vi "capture.vi"() -> ()   [LabVIEW 2014]
uses:
  <vilib>/Instr/_visa.llb/VISA Configure Serial Port (Instr).vi
panel:
  in  "stop":bool
  in  "Home":bool
  in  "error in (no error)":errorcluster
  in  "stop 2":bool
  out "x-position":dbl
  out "y-position":dbl
  out "z-position":dbl
  in  "X um":dbl
  in  "Y um":dbl
  out "error out":errorcluster
  in  "VISA resource name":refnum<visa-resource-name>
  out "y":sgl
  out "x":sgl
  out "Coordinate System Out (Set Coordinate System 1)":T1 {"Measurement System"."Axis Reference" items=["Direct", "Indirect"]; "Measurement System"."Angle (deg)" format="%.2f"; "Measurement System"."Origin"."Y" format="%.2f"; "Measurement System"."Origin"."X" format="%.2f"; "Reference System"."Axis Reference" items=["Direct", "Indirect"]; "Reference System"."Angle (deg)" format="%.2f"; "Reference System"."Origin"."Y" format="%.2f"; "Reference System"."Origin"."X" format="%.2f"}
  out "Objects (pixel) (Object Tracking 1)":T2(array[cluster])
  out "Image":T3(plugin-control)
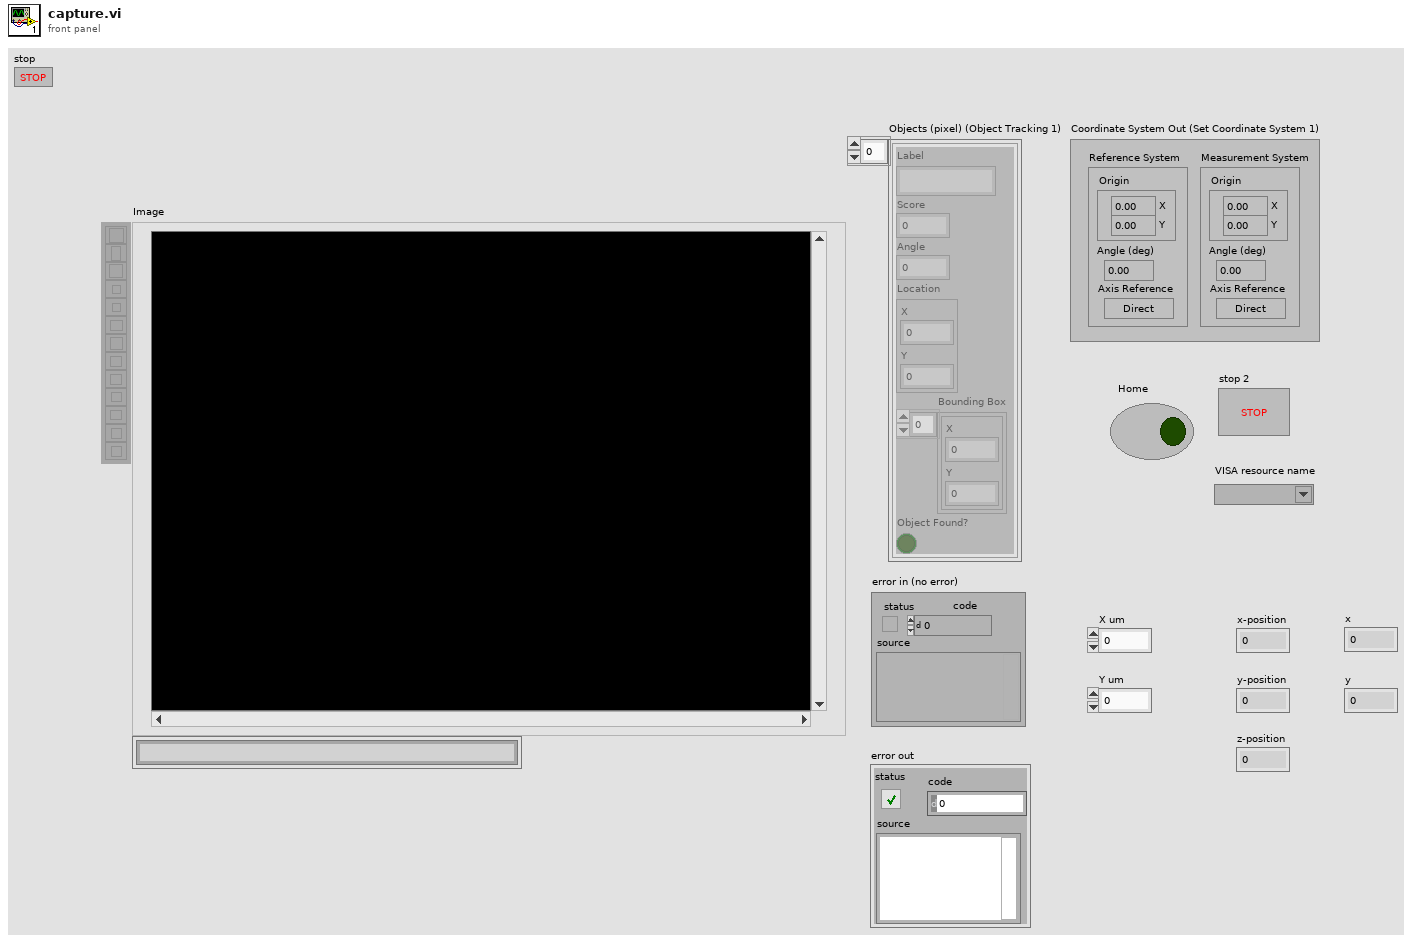
[diagram p1: front panel]
types:
  T1 = cluster{"Reference System":cluster{"Origin":cluster{"X":sgl, "Y":sgl}, "Angle (deg)":sgl, "Axis Reference":u32}, "Measurement System":cluster{"Origin":cluster{"X":sgl, "Y":sgl}, "Angle (deg)":sgl, "Axis Reference":u32}}
  T2 = cluster{"Label":string, "Score":i32, "Angle":dbl, "Location":cluster{"X":dbl, "Y":dbl}, "Bounding Box":cluster{"X":dbl, "Y":dbl}[], "Object Found?":bool}[]
  T3 = typedef "IMAQ Image.ctl" = refnum<image>
  T4 = typedef "Image Type" = u32
  T5 = cluster{"Origin":cluster{"X":sgl, "Y":sgl}, "Angle (deg)":sgl, "Axis Reference":u32}
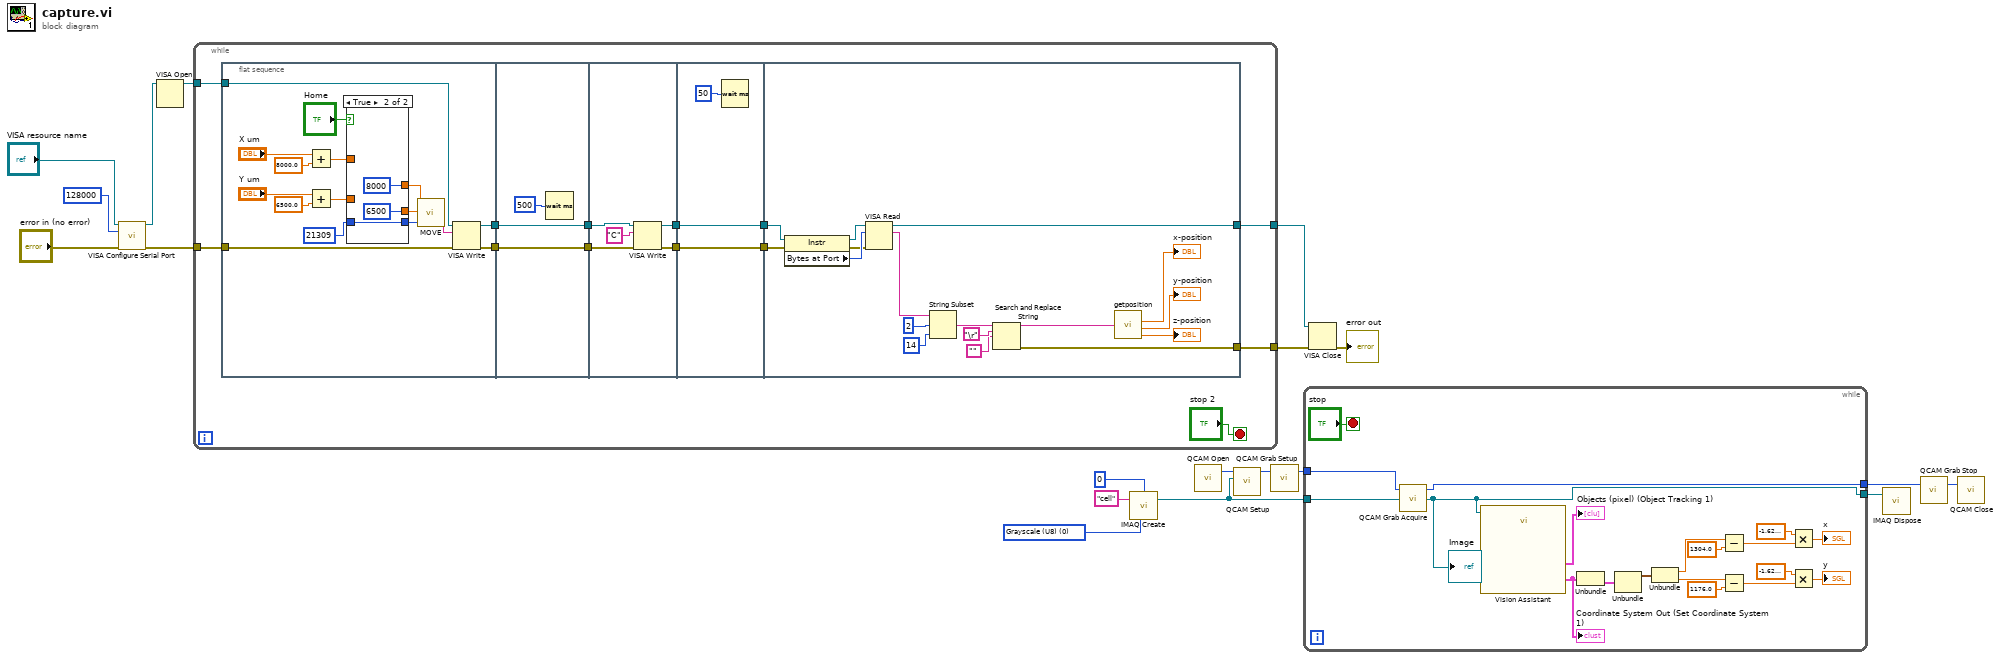
[diagram p0: block diagram]
diagram:
  w11 = T4 0 items=["Grayscale (U8)", "Grayscale (I16)", "Grayscale (SGL)", "Complex (CSG)", "RGB (U32)", "HSL (U32)", "RGB (U64)", "Grayscale (U16)"] ("Image Type")
  n1 = call-poly "VISA Configure Serial Port"("VISA resource name"="VISA resource name", "baud rate (9600)"=u32 128000, "error in (no error)"="error in (no error)") -> ("VISA resource name out"=w15:refnum<visa-resource-name>, "error out"=w17:errorcluster)  [unwired: 11 in]
  n2 = VISA Open(VISA resource name=w15) -> (VISA resource name=w3:refnum<visa-resource-name>)  [unwired: 4 in, 1 out]
  n3 = while {
    tunnel: w17 -> [w24]
    tunnel: [w23] -> w13
    tunnel: w3 -> [w22]
    tunnel: [w21] -> w2
    stop <- "stop 2" stop-if-true
    n4 = flat-sequence {
      tunnel: [w48] -> w32
      tunnel: [w47] -> w31
      tunnel: w22 -> [w43]
      tunnel: w24 -> [w42]
      tunnel: w32 -> [w57]
      tunnel: [w57] -> w30
      tunnel: [w55] -> w29
      tunnel: w31 -> [w55]
      tunnel: w30 -> [w59]
      tunnel: w29 -> [w61]
      tunnel: [w60] -> w28
      tunnel: [w58] -> w27
      tunnel: w28 -> [w65]
      tunnel: [w65] -> w26
      tunnel: [w63] -> w25
      tunnel: w27 -> [w63]
      tunnel: w26 -> [w77]
      tunnel: [w76] -> w21
      tunnel: w25 -> [w73]
      tunnel: [w71] -> w23
      frame #0 {
        n5 = Add(x="X um", y=8000.0) -> (x+y=w39:dbl)
        n6 = Add(x="Y um", y=6500.0) -> (x+y=w37:dbl)
        n7 = case shown="True" "Home" {
          tunnel: [w51 8000] -> w46
          tunnel: w39 -> [w51 _]
          tunnel: [w50 6500] -> w45
          tunnel: w37 -> [w50 _]
          tunnel: [w49 w52] -> w44
          tunnel: 21309 -> [w49 w52]
          frame False {
          }
          frame True {
          }
        }
        n8 = call "MOVE.vi"("Z"=w44, "Y"=w45, "x"=w46) -> ("MOVE COMMAND"=w35:string)
        n9 = VISA Write(VISA resource name=w43, write buffer=w35, error in (no error)=w42) -> (VISA resource name out=w47:refnum<visa-resource-name>, error out=w48:errorcluster)  [unwired: 1 out]
      }
      frame #1 {
        n10 = Wait (ms)(milliseconds to wait=u32 500) -> ()  [unwired: 1 out]
      }
      frame #2 {
        n11 = VISA Write(VISA resource name=w61, write buffer="C", error in (no error)=w59) -> (VISA resource name out=w60:refnum<visa-resource-name>, error out=w58:errorcluster)  [unwired: 1 out]
      }
      frame #3 {
        n12 = Wait (ms)(milliseconds to wait=u32 50) -> ()  [unwired: 1 out]
      }
      frame #4 {
        n13 = property class="Instr"(reference=w77, error in=w73) -> (reference out=w82:refnum<visa-resource-name>, error out=w72:errorcluster, "Bytes at Port"=w78:u32)
        n14 = VISA Read(VISA resource name=w82, byte count=w78, error in (no error)=w72) -> (VISA resource name out=w76:refnum<visa-resource-name>, read buffer=w69:string)  [unwired: 2 out]
        n15 = String Subset(string=w69, offset (0)=2, length (rest)=14 ("length (rest)")) -> (substring=w66:string)
        n16 = Search and Replace String(input string=w66, search string="\r", replace string="") -> (result string=w70:string, error out=w71:errorcluster)  [unwired: 5 in, 2 out]
        n17 = call "getposition.vi"("string"=w70) -> ("x-position"=→"x-position":dbl, "y-position"=→"y-position":dbl, "z-position"=→"z-position":dbl)  [unwired: 1 out]
      }
    }
  }
  n18 = call "IMAQ Create"("Border Size"=0, "Image Name"="cell", "Image Type"=w11) -> ("New Image"=w6:T3)  [unwired: 2 in, 1 out]
  n19 = call <userlib>:"QCAM Open.vi"() -> ("cameraId out"=w9:u32)  [unwired: 2 in, 1 out]
  n20 = call <userlib>:"QCAM Setup.vi"("Image"=w6, "cameraId"=w9) -> ("cameraId out"=w8:u32)  [unwired: 5 in, 4 out]
  n21 = call <userlib>:"QCAM Grab Setup.vi"("cameraId"=w8) -> ("cameraId out"=w7:u32)  [unwired: 1 in, 1 out]
  n22 = while {
    tunnel: w6 -> [w100]
    tunnel: w7 -> [w101]
    tunnel: [w99] -> w4
    tunnel: [w84] -> w1
    stop <- "stop" stop-if-true
    n23 = call <userlib>:"QCAM Grab Acquire.vi"("Image"=w100, "cameraId"=w101) -> ("Image Out"=w84:T3, "cameraId out"=w99:u32)  [unwired: 1 in, 1 out]
    "Image" <- w84
    n24 = call "Vision Assistant"("Image In"=w84) -> ("Objects (pixel) (Object Tracking 1)"=→"Objects (pixel) (Object Tracking 1)":T2, "Coordinate System Out (Set Coordinate System 1)"=w86:T1)  [unwired: 23 in, 2 out]
    "Coordinate System Out (Set Coordinate System 1)" <- w86
    n25 = Unbundle(w86) -> ("Measurement System"=w87:T5)  [unwired: 1 out]
    n26 = Unbundle(w87) -> ("Origin"=w88:cluster{"X":sgl, "Y":sgl})  [unwired: 2 out]
    n27 = Unbundle(w88) -> ("X"=w89:sgl, "Y"=w91:sgl)
    n28 = Subtract(x=w89, y=sgl 1304.0) -> (x-y=w93:sgl)
    n29 = Subtract(x=w91, y=sgl 1176.0) -> (x-y=w96:sgl)
    n30 = Multiply(x=sgl -1.62, y=w93) -> (x*y=→"x":sgl)
    n31 = Multiply(x=sgl -1.62, y=w96) -> (x*y=→"y":sgl)
  }
  n32 = VISA Close(VISA resource name=w2, error in (no error)=w13) -> (error out=→"error out":errorcluster)
  n33 = call "IMAQ Dispose"("Image"=w1) -> ()  [unwired: 5 in, 1 out]
  n34 = call <userlib>:"QCAM Grab Stop.vi"("cameraId"=w4) -> ("cameraId Out"=w5:u32)  [unwired: 1 in, 1 out]
  n35 = call <userlib>:"QCAM Close.vi"("cameraId"=w5) -> ()  [unwired: 2 in, 1 out]
